vi "Pre-Process.vi"(11 "TEMPLATE jettl in":refnum<class "TEMPLATE jettl.lvclass">) -> (3 "TEMPLATE jettl out":refnum<class "TEMPLATE jettl.lvclass">)   [LabVIEW 2021, in "_Template.lvlib" / "Templates.lvlib" / "TEMPLATE jettl.lvlib" / "TEMPLATE jettl.lvclass"]
uses:
  TEMPLATE jettl.lvclass
  TEMPLATE jettl.lvclass/TEMPLATE jettl.ctl
  jettl/jettl/jettl/jettl.lvclass
  jettl/Setup Msg Strategy/Setup Msg Strategy.lvlib
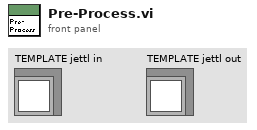
[diagram p1: front panel]
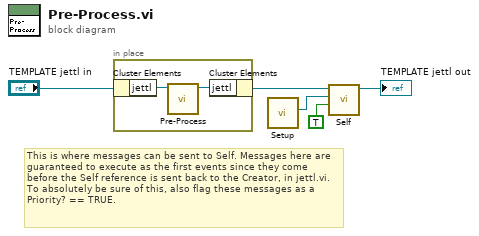
[diagram p0: block diagram]
diagram:
  # "This is where messages can be sent to Self. Messages here are guaranteed to execute as the first events since they come before the Self reference is sent back to the Creator, in jettl.vi. To absolutely be sure of this, also flag these messages as a Priority? == TRUE."
  n1 = in-place {
    n2 = in-place-cluster #1("TEMPLATE jettl in") -> ("jettl"=w7:refnum<class "jettl.lvclass">)
    n3 = call-dynamic "Pre-Process.vi"("jettl in"=w7) -> ("jettl out"=w6:refnum<class "jettl.lvclass">)  [unwired: 10 in]
    n4 = in-place-cluster #1("jettl"=w6) -> (w4:refnum<class "TEMPLATE jettl.lvclass">)
  }
  n5 = call "Setup.vi"() -> ("Msg Strategy"=w2:refnum<class "Msg Strategy.lvclass">)  [unwired: 11 in]
  n6 = call-dynamic "Self.vi"("Priority?"=TRUE, "Msg Strategy"=w2, "TEMPLATE jettl in"=w4) -> ("TEMPLATE jettl out"=→"TEMPLATE jettl out":refnum<class "TEMPLATE jettl.lvclass">)  [unwired: 8 in]
